vi "LoadVisionPanel001.vi"(8 "error in (no error)":errorcluster) -> (0 "error out":errorcluster, 2 "This VI":refnum<vi>)   [LabVIEW 2019]
uses:
  <vilib>/Utility/miscctls.llb/LVPointTypeDef.ctl
panel:
  in  "Tab Control":enum32{"視覺", "震動盤", "IO", "視覺手臂校正"}(tab)
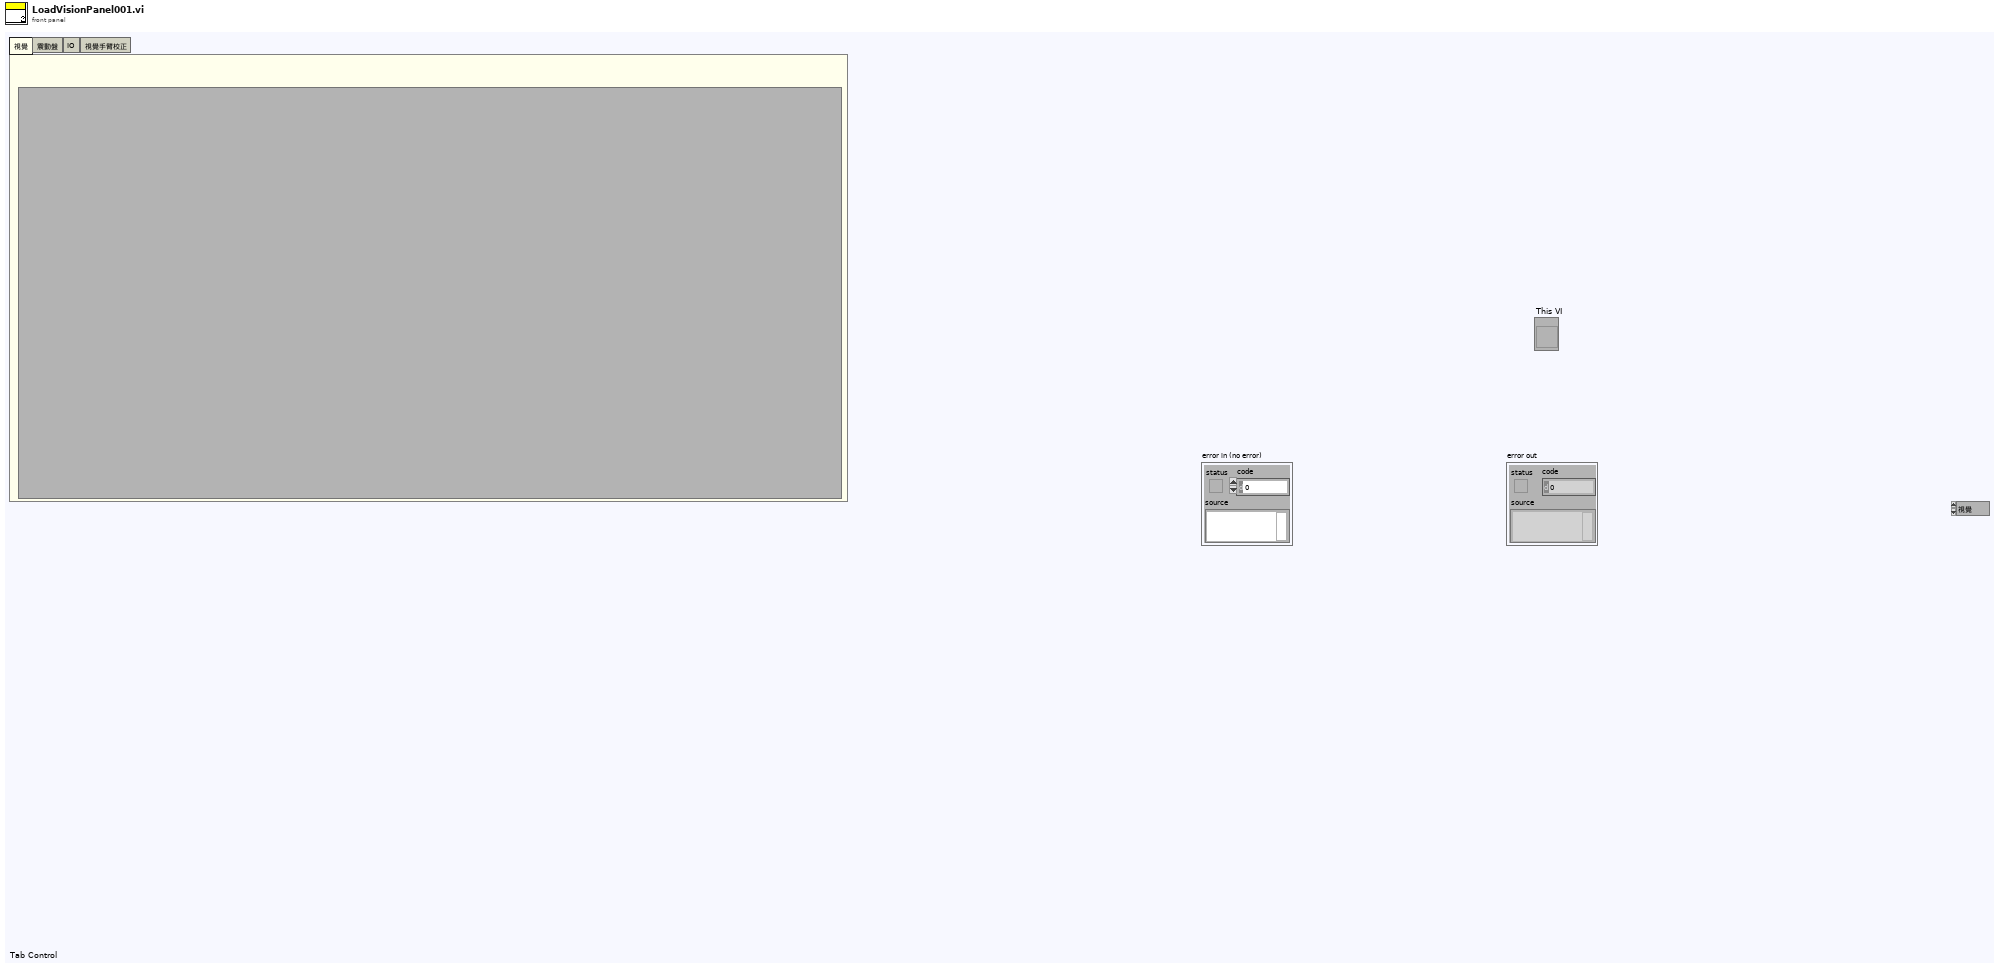
[diagram p1: front panel]
types:
  T1 = typedef "LVPointTypeDef.ctl" = cluster{"Horizontal":i16, "Vertical":i16}
  T2 = typedef "LVPositionTypeDef.ctl" = cluster{"Left":i32, "Top":i32}
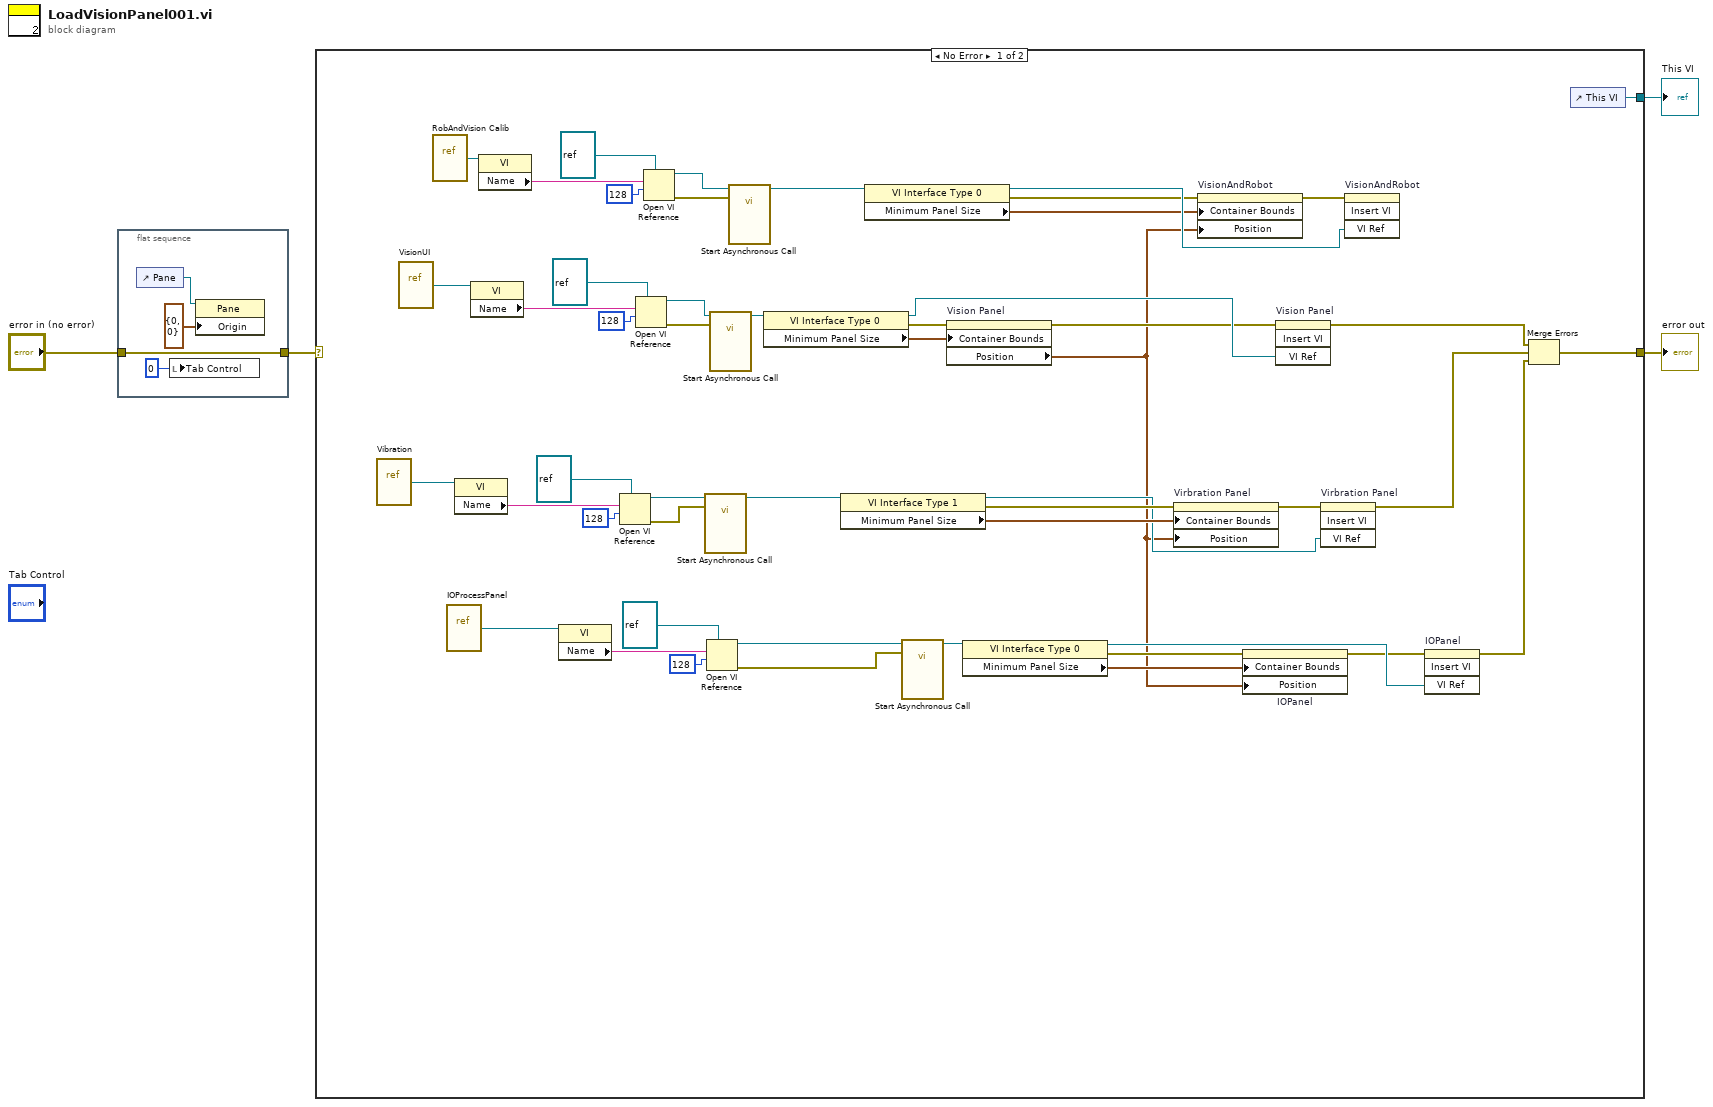
[diagram p0: block diagram]
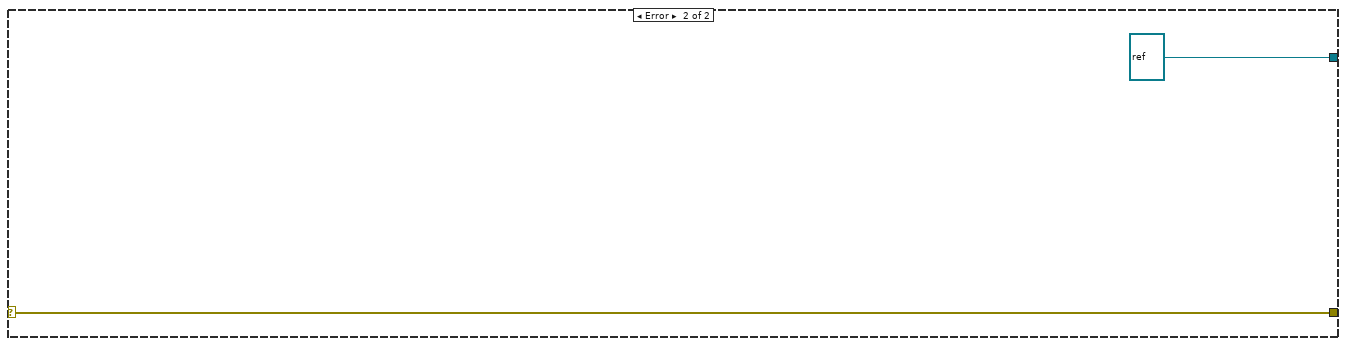
[diagram p2: hidden frame]
diagram:
  n1 = flat-sequence {
    tunnel: [w8] -> w1
    tunnel: "error in (no error)" -> [w8]
    frame #0 {
      n2 = control-ref of="Pane"() -> (w6:refnum<vi>)
      n3 = local write "Tab Control"(0) -> ()
      n4 = property class="Pane"(reference=w6, "Origin"=T1 {"Horizontal"=0, "Vertical"=0}) -> ()  [unwired: 1 in, 2 out]
    }
  }
  n5 = case shown="No Error" w1 {
    selector: w1 -> [_ w60]
    tunnel: [w52 refnum<vi> refnum ("type specifier VI Refnum (for type only)")] -> w4
    tunnel: [w23 w60] -> w3
    frame No Error {
      n6 = vi-ref "Vibration.vi"() -> (w38:refnum<vi>)
      n7 = vi-ref "VisionUI.vi"() -> (w58:refnum<vi>)
      n8 = vi-ref "RobAndVision Calib.vi"() -> (w10:refnum<vi>)
      n9 = vi-ref "IOProcessPanel.vi"() -> (w37:refnum<vi>)
      n10 = property class="VI"(reference=w38) -> ("Name"=w39:string)  [unwired: 1 in, 2 out]
      n11 = property class="VI"(reference=w58) -> ("Name"=w57:string)  [unwired: 1 in, 2 out]
      n12 = property class="VI"(reference=w10) -> ("Name"=w11:string)  [unwired: 1 in, 2 out]
      n13 = property class="VI"(reference=w37) -> ("Name"=w36:string)  [unwired: 1 in, 2 out]
      n14 = Open VI Reference(type specifier VI Refnum (for type only)=refnum<vi> refnum, vi path=w39, options=128) -> (vi reference=w41:refnum<vi>, error out=w42:errorcluster)  [unwired: 3 in]
      n15 = Open VI Reference(type specifier VI Refnum (for type only)=refnum<vi> refnum, vi path=w57, options=128) -> (vi reference=w55:refnum<vi>, error out=w54:errorcluster)  [unwired: 3 in]
      n16 = Open VI Reference(type specifier VI Refnum (for type only)=refnum<vi> refnum, vi path=w11, options=128) -> (vi reference=w13:refnum<vi>, error out=w14:errorcluster)  [unwired: 3 in]
      n17 = call-by-ref "Start Asynchronous Call"(reference=w41, error in=w42) -> (reference out=w44:refnum<vi>)  [unwired: 11 in, 2 out]
      n18 = Open VI Reference(type specifier VI Refnum (for type only)=refnum<vi> refnum, vi path=w36, options=128) -> (vi reference=w34:refnum<vi>, error out=w33:errorcluster)  [unwired: 3 in]
      n19 = call-by-ref "Start Asynchronous Call"(reference=w55, error in=w54) -> (reference out=w51:refnum<vi>)  [unwired: 12 in, 1 out]
      n20 = call-by-ref "Start Asynchronous Call"(reference=w13, error in=w14) -> (reference out=w16:refnum<vi>)  [unwired: 12 in, 1 out]
      n21 = property class="VI Interface Type 0"(reference=w51) -> (reference out=w48:refnum<vi>, error out=w49:errorcluster, "Minimum Panel Size"=w50:T1)  [unwired: 1 in]
      n22 = property class="VI Interface Type 1"(reference=w44) -> (reference out=w28:refnum<vi>, error out=w46:errorcluster, "Minimum Panel Size"=w45:T1)  [unwired: 1 in]
      n23 = property class="VI Interface Type 0"(reference=w16) -> (reference out=w19:refnum<vi>, error out=w18:errorcluster, "Minimum Panel Size"=w17:T1)  [unwired: 1 in]
      n24 = call-by-ref "Start Asynchronous Call"(reference=w34, error in=w33) -> (reference out=w31:refnum<vi>)  [unwired: 12 in, 1 out]
      n25 = property on="Vision Panel" class="SubPnl"(error in=w49, "Container Bounds"=w50) -> (error out=w47:errorcluster, "Position"=w9:T2)  [unwired: 1 in, 1 out]
      n26 = property class="VI Interface Type 0"(reference=w31) -> (reference out=w27:refnum<vi>, error out=w29:errorcluster, "Minimum Panel Size"=w30:T1)  [unwired: 1 in]
      n27 = property on="Virbration Panel" class="SubPnl"(error in=w46, "Container Bounds"=w45, "Position"=w9) -> (error out=w21:errorcluster)  [unwired: 1 in, 1 out]
      n28 = property on="VisionAndRobot" class="SubPnl"(error in=w18, "Container Bounds"=w17, "Position"=w9) -> (error out=w20:errorcluster)  [unwired: 1 in, 1 out]
      n29 = property on="IOPanel" class="SubPnl"(error in=w29, "Container Bounds"=w30, "Position"=w9) -> (error out=w22:errorcluster)  [unwired: 1 in, 1 out]
      n30 = invoke on="Vision Panel" class="SubPnl" method="Insert VI"(error in=w47, "VI Ref"=w48) -> (error out=w26:errorcluster)  [unwired: 2 in, 3 out]
      n31 = invoke on="Virbration Panel" class="SubPnl" method="Insert VI"(error in=w21, "VI Ref"=w28) -> (error out=w25:errorcluster)  [unwired: 2 in, 3 out]
      n32 = invoke on="VisionAndRobot" class="SubPnl" method="Insert VI"(error in=w20, "VI Ref"=w19) -> ()  [unwired: 2 in, 4 out]
      n33 = invoke on="IOPanel" class="SubPnl" method="Insert VI"(error in=w22, "VI Ref"=w27) -> (error out=w24:errorcluster)  [unwired: 2 in, 3 out]
      n34 = Merge Errors(w26, w25, w24) -> (w23:errorcluster)
      n35 = control-ref of="This VI"() -> (w52:refnum<vi>)
    }
    frame Error {
    }
  }
  "error out" <- w3
  "This VI" <- w4
